vi "OxITC503 _Config_ Auto-Manual.vi"(2 "error in":errorcluster, 3 "Auto Status":T1(ring), 4 "VISA session":refnum<visa-resource-name>) -> (0 "error out (no error)":errorcluster, 1 "VISA session":refnum<visa-resource-name>)   [LabVIEW 2013]
doc: "Allows the heater and gas flow control functions to be set to AUTO or MANUAL."
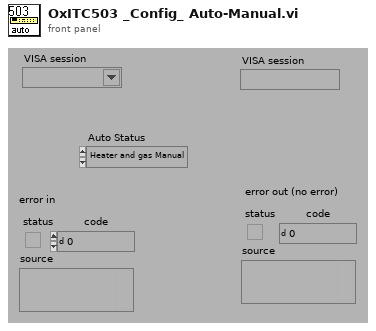
[diagram p1: front panel]
types:
  T1 = enum16{"Heater and gas Manual", "Heater Auto, Gas Manual", "Heater Manual, Gas Auto", "Heater and Gas Auto"}
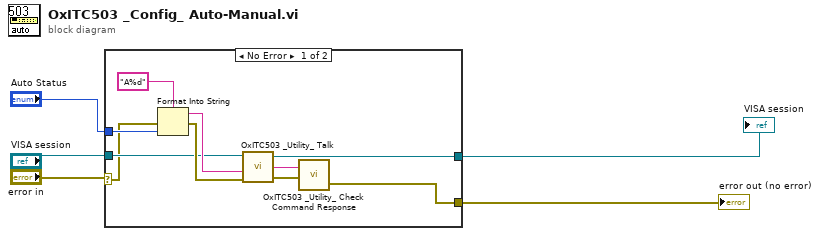
[diagram p0: block diagram]
diagram:
  n1 = case shown="No Error" "error in" {
    selector: "error in" -> [w6 w17]
    tunnel: [w12 w16] -> w5
    tunnel: "VISA session" -> [w11 w16]
    tunnel: "Auto Status" -> [w10 _]
    tunnel: [w7 w17] -> w2
    frame No Error {
      n2 = Format Into String(format string="A%d" ("Format String"), error in=w6, w10) -> (resulting string=w14:string, error out=w15:errorcluster)  [unwired: 1 in]
      n3 = call "OxITC503 _Utility_ Talk.vi"("VISA session"=w11, "Command"=w14, "error in (no error)"=w15) -> ("VISA session"=w12:refnum<visa-resource-name>, "read buffer"=w9:string, "error out (no error)"=w8:errorcluster)  [unwired: 2 in]
      n4 = call "OxITC503 _Utility_ Check Command Response.vi"("error in"=w8, "read buffer"=w9) -> ("error out (no error)"=w7:errorcluster)  [unwired: 1 out]
    }
    frame Error {
    }
  }
  "error out (no error)" <- w2
  "VISA session" <- w5
